vi "SDCP Synchronize.vi"(2 "error in (no error)":errorcluster, 3 "COM Port In":refnum<visa-resource-name>) -> (0 "error out":errorcluster, 1 "COM Port Out":refnum<visa-resource-name>)   [LabVIEW 2020]
uses:
  <vilib>/Instr/_visa.llb/VISA Flush IO Buffer Mask.ctl
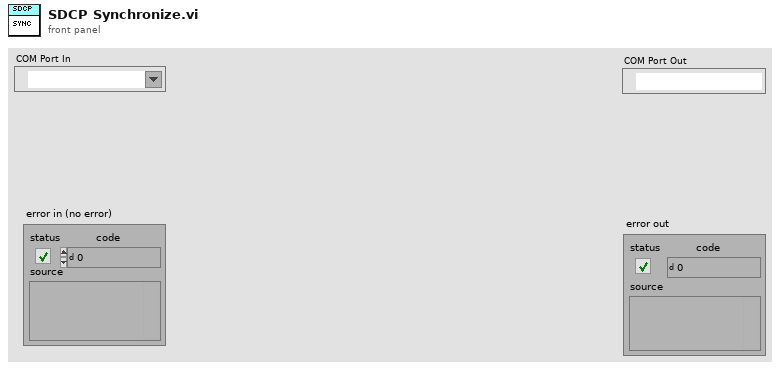
[diagram p1: front panel]
types:
  T1 = typedef "VISA Flush IO Buffer Mask.ctl" = u16
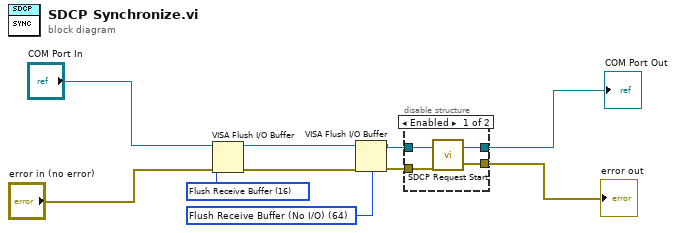
[diagram p0: block diagram]
diagram:
  w7 = T1 64 items=["Flush Receive Buffer"=16, "Write Transmit Buffer to Device"=32, "Flush Receive Buffer (No I/O)"=64, "Flush Transmit Buffer"=128] ("Mask")
  w10 = T1 16 items=["Flush Receive Buffer"=16, "Write Transmit Buffer to Device"=32, "Flush Receive Buffer (No I/O)"=64, "Flush Transmit Buffer"=128] ("Mask")
  n1 = VISA Flush I/O Buffer(VISA resource name="COM Port In", mask (16)=w10, error in (no error)="error in (no error)") -> (VISA resource name out=w8:refnum<visa-resource-name>, error out=w9:errorcluster)
  n2 = VISA Flush I/O Buffer(VISA resource name=w8, mask (16)=w7, error in (no error)=w9) -> (VISA resource name out=w6:refnum<visa-resource-name>, error out=w5:errorcluster)
  n3 = disable-structure shown="Enabled" {
    disable-tunnel: w6 -> [w14 w16]
    disable-tunnel: w5 -> [w13 w15]
    disable-tunnel: [w12 w16] -> w2
    disable-tunnel: [w11 w15] -> w3
    frame Enabled {
      n4 = call "SDCP Request Start.vi"("error in (no error)"=w13, "COM Port"=w14) -> ("error out"=w11:errorcluster, "COM Port Out"=w12:refnum<visa-resource-name>)
    }
    frame Disabled {
    }
  }
  "error out" <- w3
  "COM Port Out" <- w2
